vi "Clear Serial Port.vi"(8 "error in (no error)":errorcluster, 11 "Listener In.lvclass":refnum<class "Listener.lvclass">) -> (0 "error out":errorcluster, 3 "Listener out":refnum<class "Listener.lvclass">)   [LabVIEW 2019, in "Listener.lvclass"]
doc: "Calls Visa Clear on the specified COM port"
uses:
  Listener.lvclass
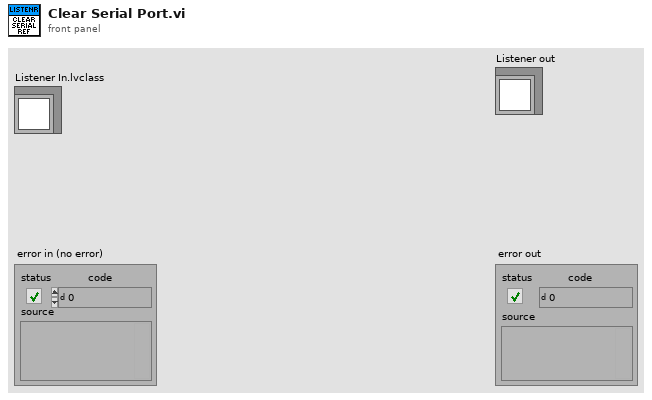
[diagram p1: front panel]
types:
  T1 = typedef "Listener.lvclass/Protocol.ctl" = enum16{"RS-XXX", "AK RS-XXX", "VISA", "TCPIP", "AK TCPIP", "UDP", "GPIB ConvBox"}
  T2 = typedef "Listener.lvclass/VISA Data Structure.ctl" = cluster{"Protocol Ref Out":refnum<visa-resource-name>, "Listener Ref Out":refnum<visa-resource-name>, "Data Length":u32, "Data":string}
  T3 = typedef "Listener.lvclass/RS-xxx To GPIB ConvBox Data Structure.ctl" = cluster{"Protocol Port Ref":refnum<visa-resource-name>, "Listener Port Ref":refnum<visa-resource-name>, "Data":string, "Command Messages Read":string[], "Address":string}
  T4 = typedef "Listener.lvclass/RS-xxx Data Structure.ctl" = cluster{"Listener Port Ref":refnum<visa-resource-name>, "Protocol Port Ref":refnum<visa-resource-name>, "Virtual COM Port Settings 1":cluster{"Port":string, "Baud Rate":u32, "Data Bits":u16, "Parity":enum16{"None", "Odd", "Even", "Mark", "Space"}, "Stop Bits":u16, "Flow Control":u16, "XON":enum16{"NUL", "SOH", "STX", "ETX", "EOT", "ENQ", "ACK", "BEL", "BS", "HT", "LF", "VT", "FF", "CR", "SO", "SI", "DLE", "DC1", "DC2", "DC3", "DC4", "NAK", "SYN", "ETB", "CAN", "EM", "SUB", "ESC", "FS", "GS", "RS", "US", "SP", "!", "\"", "#", "$", "%", "&", "'", "(", ")", "*", "+", ",", "- (-)", ".", "/", "0", "1", "2", "3", "4", "5", "6", "7", "8", "9", ":", ";", "<", "=", ">", "?", "@", "A", "B", "C", "D", "E", "F", "G", "H", "I", "J", "K", "L", "M", "N", "O", "P", "Q", "R", "S", "T", "U", "V", "W", "X", "Y", "Z", "[", "\\", "]", "^", "_", "`", "a", "b", "c", "d", "e", "f", "g", "h", "i", "j", "k", "l", "m", "n", "o", "p", "q", "r", "s", "t", "u", "v", "w", "x", "y", "z", "{", "|", "}", "~"}, "XOFF":enum16{"NUL", "SOH", "STX", "ETX", "EOT", "ENQ", "ACK", "BEL", "BS", "HT", "LF", "VT", "FF", "CR", "SO", "SI", "DLE", "DC1", "DC2", "DC3", "DC4", "NAK", "SYN", "ETB", "CAN", "EM", "SUB", "ESC", "FS", "GS", "RS", "US", "SP", "!", "\"", "#", "$", "%", "&", "'", "(", ")", "*", "+", ",", "- (-)", ".", "/", "0", "1", "2", "3", "4", "5", "6", "7", "8", "9", ":", ";", "<", "=", ">", "?", "@", "A", "B", "C", "D", "E", "F", "G", "H", "I", "J", "K", "L", "M", "N", "O", "P", "Q", "R", "S", "T", "U", "V", "W", "X", "Y", "Z", "[", "\\", "]", "^", "_", "`", "a", "b", "c", "d", "e", "f", "g", "h", "i", "j", "k", "l", "m", "n", "o", "p", "q", "r", "s", "t", "u", "v", "w", "x", "y", "z", "{", "|", "}", "~"}, "End Read on Termination Character":bool, "End Write on Termination Character":bool, "Termination Character":u8}, "Virtual COM Port Settings 2":cluster{"Port":string, "Baud Rate":u32, "Data Bits":u16, "Parity":enum16{"None", "Odd", "Even", "Mark", "Space"}, "Stop Bits":u16, "Flow Control":u16, "XON":enum16{"NUL", "SOH", "STX", "ETX", "EOT", "ENQ", "ACK", "BEL", "BS", "HT", "LF", "VT", "FF", "CR", "SO", "SI", "DLE", "DC1", "DC2", "DC3", "DC4", "NAK", "SYN", "ETB", "CAN", "EM", "SUB", "ESC", "FS", "GS", "RS", "US", "SP", "!", "\"", "#", "$", "%", "&", "'", "(", ")", "*", "+", ",", "- (-)", ".", "/", "0", "1", "2", "3", "4", "5", "6", "7", "8", "9", ":", ";", "<", "=", ">", "?", "@", "A", "B", "C", "D", "E", "F", "G", "H", "I", "J", "K", "L", "M", "N", "O", "P", "Q", "R", "S", "T", "U", "V", "W", "X", "Y", "Z", "[", "\\", "]", "^", "_", "`", "a", "b", "c", "d", "e", "f", "g", "h", "i", "j", "k", "l", "m", "n", "o", "p", "q", "r", "s", "t", "u", "v", "w", "x", "y", "z", "{", "|", "}", "~"}, "XOFF":enum16{"NUL", "SOH", "STX", "ETX", "EOT", "ENQ", "ACK", "BEL", "BS", "HT", "LF", "VT", "FF", "CR", "SO", "SI", "DLE", "DC1", "DC2", "DC3", "DC4", "NAK", "SYN", "ETB", "CAN", "EM", "SUB", "ESC", "FS", "GS", "RS", "US", "SP", "!", "\"", "#", "$", "%", "&", "'", "(", ")", "*", "+", ",", "- (-)", ".", "/", "0", "1", "2", "3", "4", "5", "6", "7", "8", "9", ":", ";", "<", "=", ">", "?", "@", "A", "B", "C", "D", "E", "F", "G", "H", "I", "J", "K", "L", "M", "N", "O", "P", "Q", "R", "S", "T", "U", "V", "W", "X", "Y", "Z", "[", "\\", "]", "^", "_", "`", "a", "b", "c", "d", "e", "f", "g", "h", "i", "j", "k", "l", "m", "n", "o", "p", "q", "r", "s", "t", "u", "v", "w", "x", "y", "z", "{", "|", "}", "~"}, "End Read on Termination Character":bool, "End Write on Termination Character":bool, "Termination Character":u8}, "Data":string, "Data Length":u32}
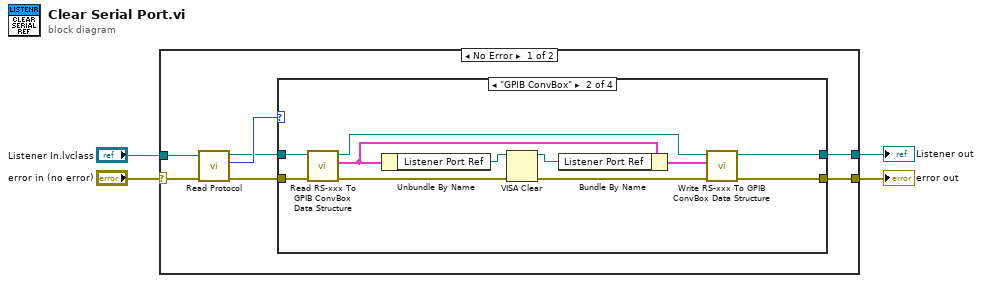
[diagram p0: block diagram]
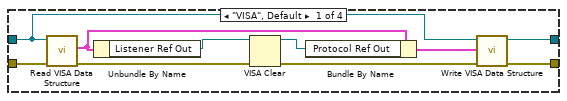
[diagram p2: hidden frame]
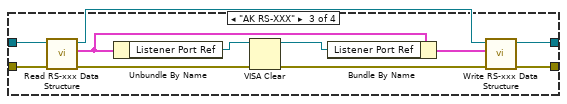
[diagram p3: hidden frame]
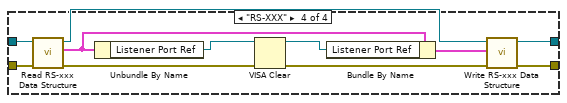
[diagram p4: hidden frame]
diagram:
  n1 = case shown="No Error" "error in (no error)" {
    selector: "error in (no error)" -> [w8 w56]
    tunnel: [w6 w56] -> w3
    tunnel: "Listener In.lvclass" -> [w11 w55]
    tunnel: [w5 w55] -> w1
    frame No Error {
      n2 = call-dynamic "Read Protocol.vi"("error in (no error)"=w8, "Listener in"=w11) -> ("error out"=w7:errorcluster, "Protocol"=w10:T1, "Listener out"=w9:refnum<class "Listener.lvclass">)  [unwired: 7 in]
      n3 = case shown="\"GPIB ConvBox\"" w10 {
        tunnel: w9 -> [w14 w32 w42 w51]
        tunnel: w7 -> [w21 w31 w41 w53]
        tunnel: [w12 w22 w38 w47] -> w6
        tunnel: [w13 w23 w33 w48] -> w5
        frame "VISA", Default {
          n4 = call-dynamic "Read VISA Data Structure.vi"("error in (no error)"=w21, "Listener in"=w14) -> ("error out"=w19:errorcluster, "VISA Data Structure"=w17:T2)  [unwired: 7 in, 1 out]
          n5 = Unbundle By Name(w17) -> ("Listener Ref Out"=w20:refnum<visa-resource-name>)
          n6 = VISA Clear(VISA resource name=w20, error in (no error)=w19) -> (VISA resource name out=w16:refnum<visa-resource-name>, error out=w18:errorcluster)
          n7 = Bundle By Name(cluster=w17, "Protocol Ref Out"=w16) -> (w15:T2)
          n8 = call-dynamic "Write VISA Data Structure.vi"("error in (no error)"=w18, "VISA Data Structure"=w15, "Listener in"=w14) -> ("error out"=w12:errorcluster, "Listener out"=w13:refnum<class "Listener.lvclass">)  [unwired: 7 in]
        }
        frame "GPIB ConvBox" {
          n9 = call-dynamic "Read RS-xxx To GPIB ConvBox Data Structure.vi"("error in (no error)"=w31, "Listener in"=w32) -> ("error out"=w30:errorcluster, "RS-xxx To GPIB ConvBox Data Structure"=w27:T3, "Listener out"=w24:refnum<class "Listener.lvclass">)  [unwired: 7 in]
          n10 = Unbundle By Name(w27) -> ("Listener Port Ref"=w29:refnum<visa-resource-name>)
          n11 = VISA Clear(VISA resource name=w29, error in (no error)=w30) -> (VISA resource name out=w26:refnum<visa-resource-name>, error out=w28:errorcluster)
          n12 = Bundle By Name(cluster=w27, "Listener Port Ref"=w26) -> (w25:T3)
          n13 = call-dynamic "Write RS-xxx To GPIB ConvBox Data Structure.vi"("error in (no error)"=w28, "RS-xxx To GPIB ConvBox Data Structure"=w25, "Listener in"=w24) -> ("error out"=w22:errorcluster, "Listener out"=w23:refnum<class "Listener.lvclass">)  [unwired: 7 in]
        }
        frame "AK RS-XXX" {
          n14 = call-dynamic "Read RS-xxx Data Structure.vi"("error in (no error)"=w41, "Listener in"=w42) -> ("error out"=w40:errorcluster, "RS-xxx Data Structure"=w36:T4, "Listener out"=w37:refnum<class "Listener.lvclass">)  [unwired: 7 in]
          n15 = Unbundle By Name(w36) -> ("Listener Port Ref"=w43:refnum<visa-resource-name>)
          n16 = VISA Clear(VISA resource name=w43, error in (no error)=w40) -> (VISA resource name out=w34:refnum<visa-resource-name>, error out=w39:errorcluster)
          n17 = Bundle By Name(cluster=w36, "Listener Port Ref"=w34) -> (w35:T4)
          n18 = call-dynamic "Write RS-xxx Data Structure.vi"("error in (no error)"=w39, "RS-xxx Data Structure"=w35, "Listener in"=w37) -> ("error out"=w38:errorcluster, "Listener out"=w33:refnum<class "Listener.lvclass">)  [unwired: 7 in]
        }
        frame "RS-XXX" {
          n19 = call-dynamic "Read RS-xxx Data Structure.vi"("error in (no error)"=w53, "Listener in"=w51) -> ("error out"=w52:errorcluster, "RS-xxx Data Structure"=w46:T4, "Listener out"=w50:refnum<class "Listener.lvclass">)  [unwired: 7 in]
          n20 = Unbundle By Name(w46) -> ("Listener Port Ref"=w54:refnum<visa-resource-name>)
          n21 = VISA Clear(VISA resource name=w54, error in (no error)=w52) -> (VISA resource name out=w45:refnum<visa-resource-name>, error out=w49:errorcluster)
          n22 = Bundle By Name(cluster=w46, "Listener Port Ref"=w45) -> (w44:T4)
          n23 = call-dynamic "Write RS-xxx Data Structure.vi"("error in (no error)"=w49, "RS-xxx Data Structure"=w44, "Listener in"=w50) -> ("error out"=w47:errorcluster, "Listener out"=w48:refnum<class "Listener.lvclass">)  [unwired: 7 in]
        }
      }
    }
    frame Error {
    }
  }
  "error out" <- w3
  "Listener out" <- w1
